vi "Lidar Subsystem.vi"() -> ()   [LabVIEW 2016]
uses:
  Lidar Global.vi
  <vilib>/Rock Robotics/Network Tables/NT Write Number.vi
panel:
  out "distance (cm)":u16
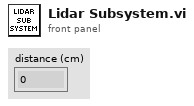
[diagram p1: front panel]
types:
  T1 = typedef "WPI_I2CDevRef.ctl" = cluster{"DevStatus":errorcluster, "Device Address":u8, "Handle":i32, "I2C Bus":T2}
  T2 = typedef "i2c_bus.ctl" = enum16{"I2C On-Board", "I2C MXP", "Invalid"}
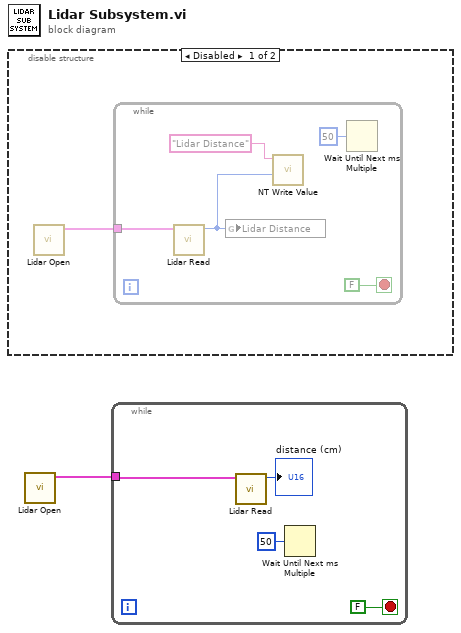
[diagram p0: block diagram]
diagram:
  n1 = disable-structure shown="Disabled" {
    frame Disabled {
      n2 = call "Lidar Open.vi"() -> ("I2CDevRef"=w2:T1)  [unwired: 11 in]
      n3 = while {
        tunnel: w2 -> [w7]
        stop <- FALSE stop-if-true
        n4 = call "Lidar Read.vi"("I2CDevRef"=w7) -> ("distance (cm)"=w4:u16)  [unwired: 10 in]
        n5 = global write "Lidar Global.vi" "Lidar Distance"(w4) -> ()
        n6 = call-poly <vilib>:"NT Write Value.vi"("Numeric"=w4, "Name"="Lidar Distance") -> ()  [unwired: 9 in, 1 out]
        n7 = Wait Until Next ms Multiple(millisecond multiple=u32 50 ("milliseconds to wait")) -> ()  [unwired: 1 out]
      }
    }
    frame Enabled {
    }
  }
  n8 = call "Lidar Open.vi"() -> ("I2CDevRef"=w1:T1)  [unwired: 11 in]
  n9 = while {
    tunnel: w1 -> [w9]
    stop <- FALSE stop-if-true
    n10 = call "Lidar Read.vi"("I2CDevRef"=w9) -> ("distance (cm)"=→"distance (cm)":u16)  [unwired: 10 in]
    n11 = Wait Until Next ms Multiple(millisecond multiple=u32 50 ("milliseconds to wait")) -> ()  [unwired: 1 out]
  }
